vi "Add State(s) to Queue__JKI_lib_State_Machine_ACBMOD.vi"(0 "State(s) in Front (\"\")":string, 5 "State(s) in (\"\")":string, 7 "State(s) at Back (\"\")":string) -> (6 "States Out":string)   [LabVIEW 2015]
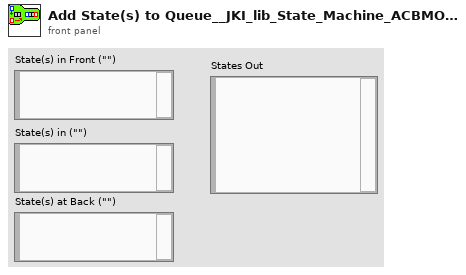
[diagram p1: front panel]
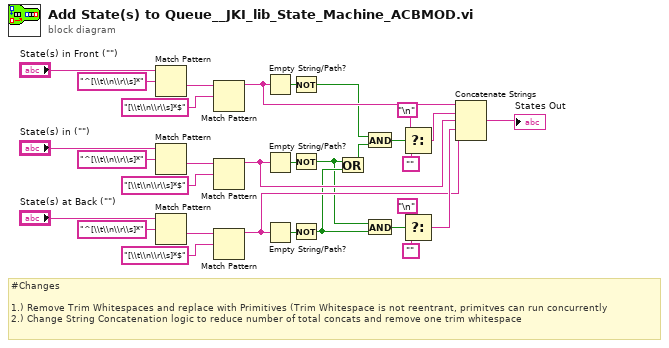
[diagram p0: block diagram]
diagram:
  # "#Changes\n\n1.) Remove Trim Whitespaces and replace with Primitives (Trim Whitespace is not reentrant, primitves can run concurrently\n2.) Change String Concatenation logic to reduce number of total concats and remove one trim whitespace"
  n1 = Match Pattern(string="State(s) in Front (\"\")", regular expression="^[\\t\\n\\r\\s]*") -> (after substring=w30:string)  [unwired: 1 in, 3 out]
  n2 = Match Pattern(string="State(s) in (\"\")", regular expression="^[\\t\\n\\r\\s]*") -> (after substring=w27:string)  [unwired: 1 in, 3 out]
  n3 = Match Pattern(string="State(s) at Back (\"\")", regular expression="^[\\t\\n\\r\\s]*") -> (after substring=w24:string)  [unwired: 1 in, 3 out]
  n4 = Match Pattern(string=w30, regular expression="[\\t\\n\\r\\s]*$") -> (before substring=w16:string)  [unwired: 1 in, 3 out]
  n5 = Match Pattern(string=w27, regular expression="[\\t\\n\\r\\s]*$") -> (before substring=w9:string)  [unwired: 1 in, 3 out]
  n6 = Match Pattern(string=w24, regular expression="[\\t\\n\\r\\s]*$") -> (before substring=w5:string)  [unwired: 1 in, 3 out]
  n7 = Empty String/Path?(string/path=w16) -> (empty?=w17:bool)
  n8 = Empty String/Path?(string/path=w9) -> (empty?=w18:bool)
  n9 = Empty String/Path?(string/path=w5) -> (empty?=w19:bool)
  n10 = Not(x=w17) -> (.not. x?=w14:bool)
  n11 = Not(x=w18) -> (.not. x?=w1:bool)
  n12 = Not(x=w19) -> (.not. x?=w2:bool)
  n13 = Or(x=w1, y=w2) -> (x .or. y?=w15:bool)
  n14 = And(x=w14, y=w15) -> (x .and. y?=w13:bool)
  n15 = And(x=w1, y=w2) -> (x .and. y?=w3:bool)
  n16 = Select(t="\n", s=w13, f="") -> (s? t:f=w12:string)
  n17 = Select(t="\n", s=w3, f="") -> (s? t:f=w6:string)
  n18 = Concatenate Strings(w16, w12, w9, w6, w5) -> (→"States Out":string)
